vi "Set velocity.vi"(0 "Zaber in":T1={"Serial port handle"="", "Axis"="", "Controller #"=0, "Min position"=0.0, "Max position"=0.0, "Min velocity"=0.0, "Max velocity"=0.0, "Firmware"="", "Device ID"=0, "Variable event"=refnum, "Variable ref"=refnum, "Resolution, usteps/step"=0, "Serial port semaphore"=refnum, "Joystick buttons"={"MinDir"=1, "MaxDir"=2, "MedSpeed"=5, "HighSpeed"=6}} {"Joystick buttons"."HighSpeed" min=1 max=25 step=1; "Joystick buttons"."MedSpeed" min=1 max=25 step=1; "Joystick buttons"."MaxDir" min=1 max=25 step=1; "Joystick buttons"."MinDir" min=1 max=25 step=1}, 2 "Velocity, mm/s":dbl, 5 "error in":errorcluster) -> (14 "Zaber out":T1={"Serial port handle"="", "Axis"="", "Controller #"=0, "Min position"=0.0, "Max position"=0.0, "Min velocity"=0.0, "Max velocity"=0.0, "Firmware"="", "Device ID"=0, "Variable event"=refnum, "Variable ref"=refnum, "Resolution, usteps/step"=0, "Serial port semaphore"=refnum, "Joystick buttons"={"MinDir"=1, "MaxDir"=2, "MedSpeed"=5, "HighSpeed"=6}} {"Joystick buttons"."HighSpeed" min=1 max=25 step=1; "Joystick buttons"."MedSpeed" min=1 max=25 step=1; "Joystick buttons"."MaxDir" min=1 max=25 step=1; "Joystick buttons"."MinDir" min=1 max=25 step=1}, 16 "Velocity, mm/s":dbl, 19 "error out":errorcluster)   [LabVIEW 2018]
uses:
  Zaber.ctl
  GenericDataEvent/GenericEvent.ctl
  ZaberVariables.ctl
  CommandZaber.ctl
  GenericDataEvent/GenericData.ctl
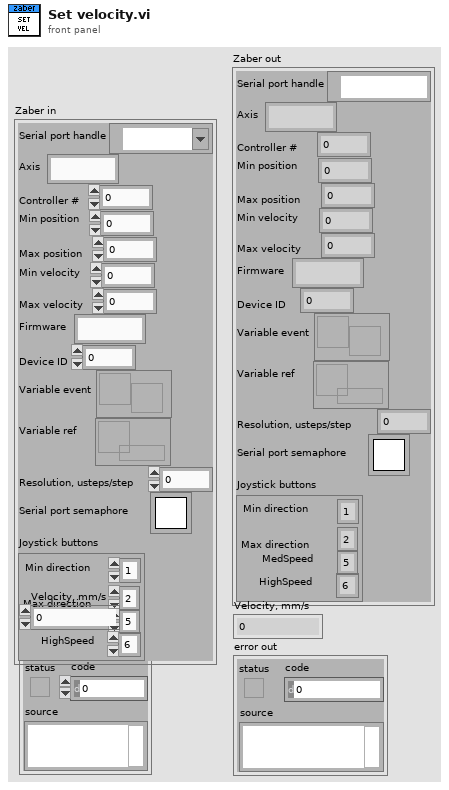
[diagram p1: front panel]
types:
  T1 = typedef "Zaber.ctl" = cluster{"Serial port handle":refnum<visa-resource-name>, "Axis":string, "Controller #":u8, "Min position":dbl, "Max position":dbl, "Min velocity":dbl, "Max velocity":dbl, "Firmware":string, "Device ID":i32, "Variable event":T2, "Variable ref":refnum<data-value>, "Resolution, usteps/step":i32, "Serial port semaphore":T3, "Joystick buttons":cluster{"MinDir":i32, "MaxDir":i32, "MedSpeed":i32, "HighSpeed":i32}}
  T2 = typedef "GenericEvent.ctl" = refnum<user-event>
  T3 = typedef "Semaphore RefNum" = refnum<k1>
  T4 = typedef "CommandZaber.ctl" = cluster{"Command":u8, "Data":i32}
  T5 = typedef "ZaberVariables.ctl" = cluster{"Position":i32, "Speed":i32, "Min soft position":dbl, "Max soft position":dbl, "Accelaration":i32}
  T6 = typedef "GenericData.ctl" = cluster{"Name":string, "Data":variant}
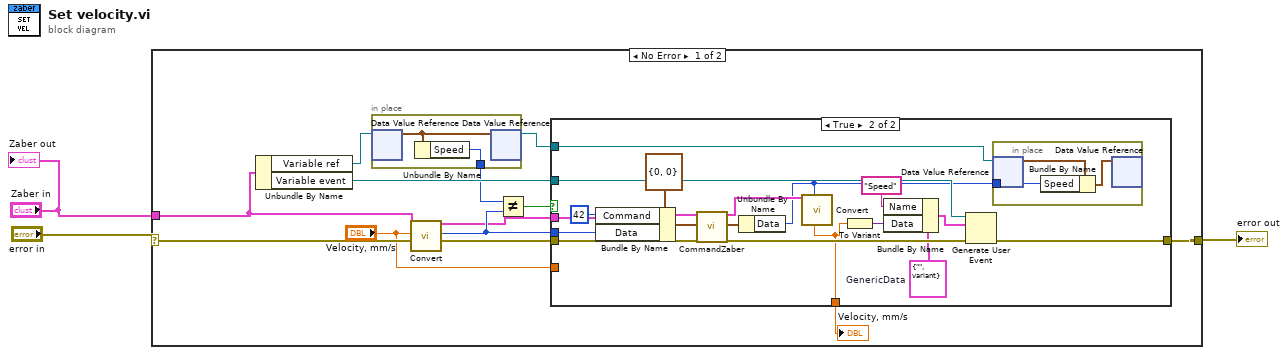
[diagram p0: block diagram]
diagram:
  n1 = case shown="No Error" "error in" {
    selector: "error in" -> [w15 w41]
    tunnel: [w14 w41] -> w2
    tunnel: "Zaber in" -> [w8 _]
    frame No Error {
      n2 = Unbundle By Name(w8) -> ("Variable ref"=w10:refnum<data-value>, "Variable event"=w13:T2)
      n3 = in-place {
        in-place-border: [w16] -> w11
        n4 = in-place-dvr #1(w10) -> (w17:T5)  [unwired: 1 out]
        n5 = Unbundle By Name(w17) -> ("Speed"=w16:i32)
        n6 = in-place-dvr #1(w17) -> (w9:refnum<data-value>)  [unwired: 1 out]
      }
      n7 = call "Convert.vi"("Zaber"=w8, "Velocity, mm/s"="Velocity, mm/s") -> ("Zaber out"=w6:T1, "Velocity, counts"=w7:i32)  [unwired: 9 in, 7 out]
      n8 = Not Equal?(x=w11, y=w7) -> (x != y?=w12:bool)
      n9 = case shown="True" w12 {
        tunnel: w15 -> [w19 w34]
        tunnel: w6 -> [_ w32]
        tunnel: w7 -> [_ w31]
        tunnel: [w19 w24] -> w14
        tunnel: w13 -> [_ w29]
        tunnel: w9 -> [_ w23]
        tunnel: [w18 w20] -> w5
        tunnel: "Velocity, mm/s" -> [w18 _]
        frame False {
        }
        frame True {
          w28 = T6 {"Name"="", "Data"=variant}  # GenericData
          n10 = Bundle By Name(cluster=T4 {"Command"=0, "Data"=0} ("Command"), "Command"=u8 42, "Data"=w31) -> (w35:T4)
          n11 = call "CommandZaber.vi"("Zaber"=w32, "Command"=w35, "error in"=w34) -> ("Zaber out"=w22:T1, "Answer"=w33:T4, "error out"=w30:errorcluster)  [unwired: 13 in, 1 out]
          n12 = Unbundle By Name(w33) -> ("Data"=w21:i32)
          n13 = call "Convert.vi"("Zaber"=w22, "Velocity, counts"=w21) -> ("Velocity, mm/s"=w20:dbl)  [unwired: 9 in, 8 out]
          n14 = To Variant(anything=w20) -> (Variant=w27:variant)
          n15 = Bundle By Name(cluster=w28, "Name"="Speed", "Data"=w27) -> (w25:T6)
          n16 = Generate User Event(user event=w29, event data cluster=w25, error in=w30) -> (error out=w24:errorcluster)  [unwired: 1 in, 1 out]
          n17 = in-place {
            in-place-border: w21 -> [w40]
            n18 = in-place-dvr #2(w23) -> (w39:T5)  [unwired: 1 out]
            n19 = Bundle By Name(cluster=w39, "Speed"=w40) -> (w38:T5)
            n20 = in-place-dvr #2(w38) -> ()  [unwired: 2 out]
          }
        }
      }
      "Velocity, mm/s" <- w5
    }
    frame Error {
    }
  }
  "error out" <- w2
  "Zaber out" <- "Zaber in"
